vi "Filter Controls and Indicators.vi"(8 "error in":errorcluster, 11 "Ctrls[]":refnum<vi>[](array[refnum])) -> (0 "error out":errorcluster, 2 "Controls":refnum<vi>[](array[refnum]), 3 "Indicators":refnum<vi>[](array[refnum]))   [LabVIEW 2013]
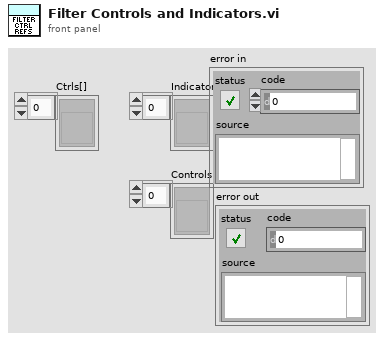
[diagram p1: front panel]
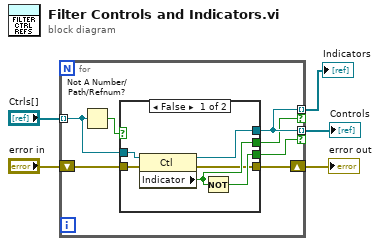
[diagram p0: block diagram]
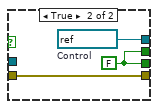
[diagram p2: hidden frame]
diagram:
  n1 = for {
    tunnel: "Ctrls[]" -> [w7] mode=indexing
    shift-right: [w8] -> w3
    shift-left: "error in" -> [w12]
    tunnel: [w11] -> w2 mode=indexing if=w9
    tunnel: [w11] -> w1 mode=indexing if=w10
    n2 = Not A Number/Path/Refnum?(number/path/refnum=w7) -> (NaN/Path/Refnum?=w6:bool)
    n3 = case shown="False" w6 {
      tunnel: w7 -> [w18 _]
      tunnel: w12 -> [w17 w21]
      tunnel: [w16 w19] -> w11
      tunnel: [w15 w20] -> w10
      tunnel: [w14 w20] -> w9
      tunnel: [w13 w21] -> w8
      frame False {
        n4 = property class="Ctl"(reference=w18, error in=w17) -> (reference out=w16:refnum<vi>, error out=w13:errorcluster, "Indicator"=w14:bool)
        n5 = Not(x=w14) -> (.not. x?=w15:bool)
      }
      frame True {
        w19 = refnum<vi> refnum  # Control
        w20 = FALSE ("Indicator")
      }
    }
  }
  "Controls" <- w1
  "Indicators" <- w2
  "error out" <- w3
